vi "Set Difference.vi"(10 "b":string[](array[string]), 11 "a":string[](array[string])) -> (2 "b - a":string[](array[string]), 3 "a - b":string[](array[string]))   [LabVIEW 2017]
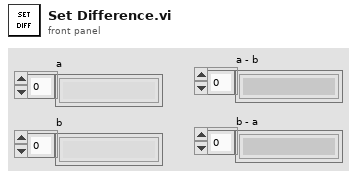
[diagram p1: front panel]
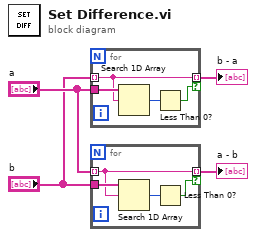
[diagram p0: block diagram]
diagram:
  n1 = for {
    tunnel: "b" -> [w7] mode=indexing
    tunnel: "a" -> [w8]
    tunnel: [w7] -> w1 mode=indexing if=w5
    n2 = Search 1D Array(1D array=w8, element=w7) -> (index of element=w6:i32)  [unwired: 1 in]
    n3 = Less Than 0?(x=w6) -> (x < 0?=w5:bool)
  }
  "b - a" <- w1
  n4 = for {
    tunnel: "a" -> [w11] mode=indexing
    tunnel: "b" -> [w12]
    tunnel: [w11] -> w4 mode=indexing if=w9
    n5 = Search 1D Array(1D array=w12, element=w11) -> (index of element=w10:i32)  [unwired: 1 in]
    n6 = Less Than 0?(x=w10) -> (x < 0?=w9:bool)
  }
  "a - b" <- w4
